vi "冰箱参数配置.vi"() -> ()   [LabVIEW 2016, in "环境动力监测库.lvlib"]
uses:
  <vilib>/Utility/config.llb/NI_LVConfig.lvlib
panel:
  in  "关闭时间":u16(ring)=2 items=["00H", "01H", "02H", "03H", "04H", "05H", "06H", "07H", "08H", "09H", "10H", "11H", "12H", "13H", "14H", "15H", "16H", "17H", "18H", "19H", "20H", "21H", "22H", "23H", "关闭"]
  in  "功能开关":enum16{"关闭", "开启"}(ring) caption="自动开关"
  in  "开启时间":u16(ring)=2 items=["00H", "01H", "02H", "03H", "04H", "05H", "06H", "07H", "08H", "09H", "10H", "11H", "12H", "13H", "14H", "15H", "16H", "17H", "18H", "19H", "20H", "21H", "22H", "23H", "关闭"]
  # "冰箱参数配置"
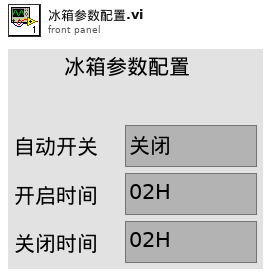
[diagram p1: front panel]
types:
  T1 = typedef "NI_LVConfig.lvlib/Config Data RefNum.ctl" = refnum<k1>
  T2 = cluster{"功能开关":enum16{"关闭", "开启"}, "开启时间":u16, "关闭时间":u16}
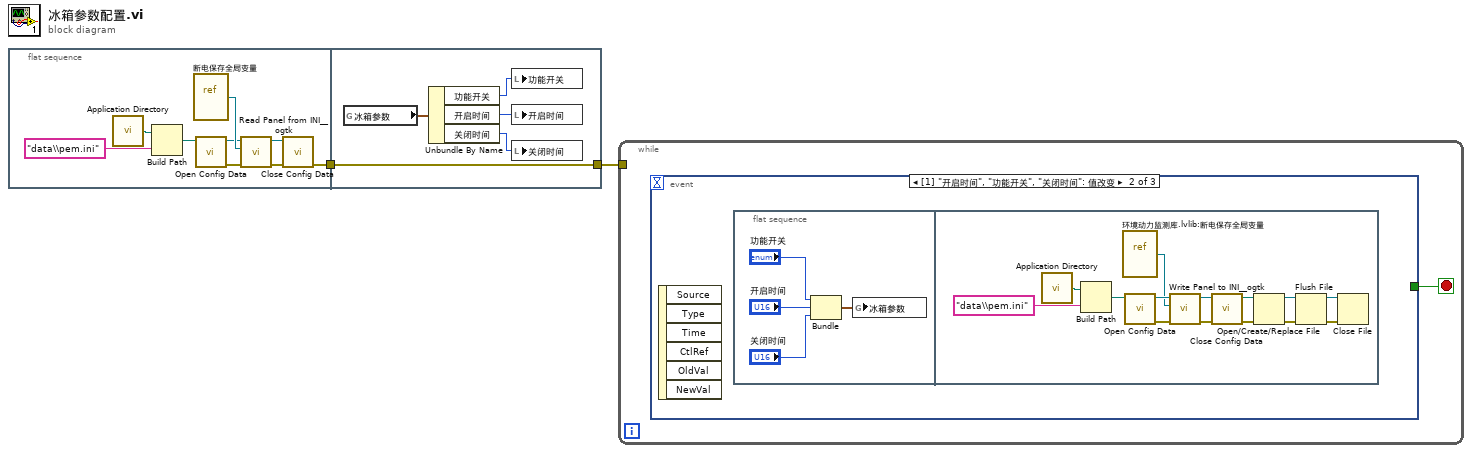
[diagram p0: block diagram]
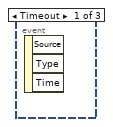
[diagram p2: hidden frame]
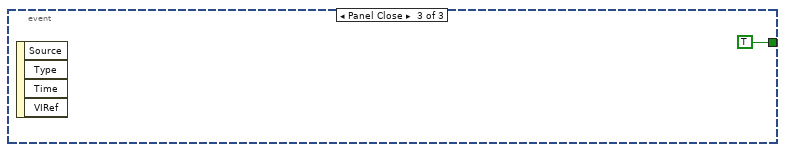
[diagram p3: hidden frame]
diagram:
  n1 = flat-sequence {
    tunnel: [w3] -> w2
    tunnel: [w16] -> w1
    tunnel: w2 -> [w16]
    frame #0 {
      n2 = call <vilib>:"Application Directory.vi"() -> ("Application Directory"=w4:path)
      n3 = Build Path(base path=w4, name or relative path="data\\pem.ini" ("名称或相对路径")) -> (appended path=w6:path)
      n4 = vi-ref "断电保存全局变量.vi"() -> (w8:refnum<vi>)
      n5 = call <vilib>:"Open Config Data.vi"("configuration file path"=w6) -> ("error out"=w10:errorcluster, "refnum"=w7:T1)  [unwired: 8 in, 1 out]
      n6 = call <userlib>:"Read Panel from INI__ogtk.vi"("error in (no error)"=w10, "VI ref"=w8, "refnum"=w7) -> ("error out"=w11:errorcluster, "refnum out"=w9:T1)  [unwired: 7 in]
      n7 = call <vilib>:"Close Config Data.vi"("error in (no error)"=w11, "refnum"=w9) -> ("error out"=w3:errorcluster)  [unwired: 8 in, 1 out]
    }
    frame #1 {
      n8 = global read "断电保存全局变量.vi" "冰箱参数"() -> (w15:T2)
      n9 = Unbundle By Name(w15) -> ("功能开关"=w14:enum16{"关闭", "开启"}, "开启时间"=w13:u16, "关闭时间"=w12:u16)
      n10 = local write "功能开关"(w14) -> ()
      n11 = local write "开启时间"(w13) -> ()
      n12 = local write "关闭时间"(w12) -> ()
    }
  }
  n13 = while {
    tunnel: w1 -> [_]
    stop <- w17 stop-if-true
    n14 = event shown="[1] \"开启时间\", \"功能开关\", \"关闭时间\": 值改变" {
      selector: _ -> [_ _ _]
      dyn-events: _ -> [_ _ _]
      timeout: _ -> [_ _ _]
      tunnel: [_ _ TRUE] -> w17
      event Timeout {
        n15 = event-data() -> ()  [unwired: 1 in, 3 out]
      }
      event "开启时间", "功能开关", "关闭时间": Value Change {
        n16 = event-data() -> ()  [unwired: 1 in, 6 out]
        n17 = flat-sequence {
          frame #0 {
            n18 = Bundle("功能开关"="功能开关", "开启时间"="开启时间", "关闭时间"="关闭时间") -> (w21:T2)  [unwired: 1 in]
            n19 = global write "断电保存全局变量.vi" "冰箱参数"(w21) -> ()
          }
          frame #1 {
            n20 = call <vilib>:"Application Directory.vi"() -> ("Application Directory"=w35:path)
            n21 = Build Path(base path=w35, name or relative path="data\\pem.ini" ("名称或相对路径")) -> (appended path=w33:path)
            n22 = vi-ref "环境动力监测库.lvlib:断电保存全局变量.vi"() -> (w31:refnum<vi>)
            n23 = call <vilib>:"Open Config Data.vi"("configuration file path"=w33) -> ("error out"=w29:errorcluster, "refnum"=w32:T1)  [unwired: 8 in, 1 out]
            n24 = call <userlib>:"Write Panel to INI__ogtk.vi"("error in (no error)"=w29, "VI ref"=w31, "refnum"=w32) -> ("error out"=w28:errorcluster, "refnum out"=w30:T1)  [unwired: 7 in]
            n25 = call <vilib>:"Close Config Data.vi"("error in (no error)"=w28, "refnum"=w30) -> ("error out"=w23:errorcluster, "file path"=w22:path)  [unwired: 8 in]
            n26 = Open/Create/Replace File(file path (use dialog)=w22, error in=w23) -> (refnum out=w26:refnum<file>, error out=w27:errorcluster)  [unwired: 4 in, 1 out]
            n27 = Flush File(refnum=w26, error in=w27) -> (refnum out=w25:refnum<file>, error out=w24:errorcluster)
            n28 = Close File(refnum=w25, error in=w24) -> ()  [unwired: 2 out]
          }
        }
      }
      event Panel Close {
        n29 = event-data() -> ()  [unwired: 1 in, 4 out]
      }
    }
  }
